vi "DecodeTDCData.vi"(11 "Buff":u32[](array[numeric])) -> (0 "Event Counter":u32, 2 "Error Read Value":u32 format="%.0x", 3 "Array":T1(array[cluster]))   [LabVIEW 2014]
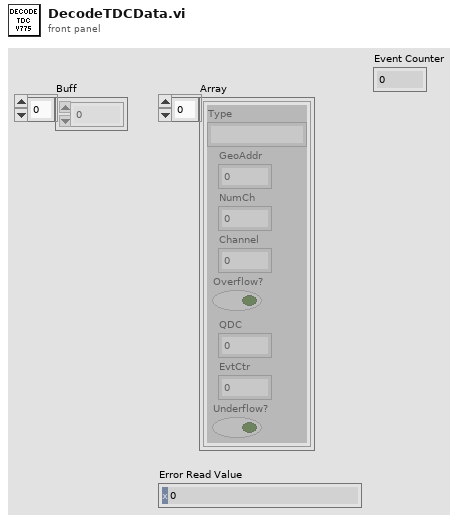
[diagram p1: front panel]
types:
  T1 = cluster{"Type":string, "GeoAddr":u8, "NumCh":u8, "Channel":u8, "Overflow?":bool, "QDC":u16, "EvtCtr":u32, "Underflow?":bool}[]
  T2 = cluster{"Type":string, "GeoAddr":u8, "NumCh":u8, "Channel":u8, "Overflow?":bool, "QDC":u16, "EvtCtr":u32, "Underflow?":bool}
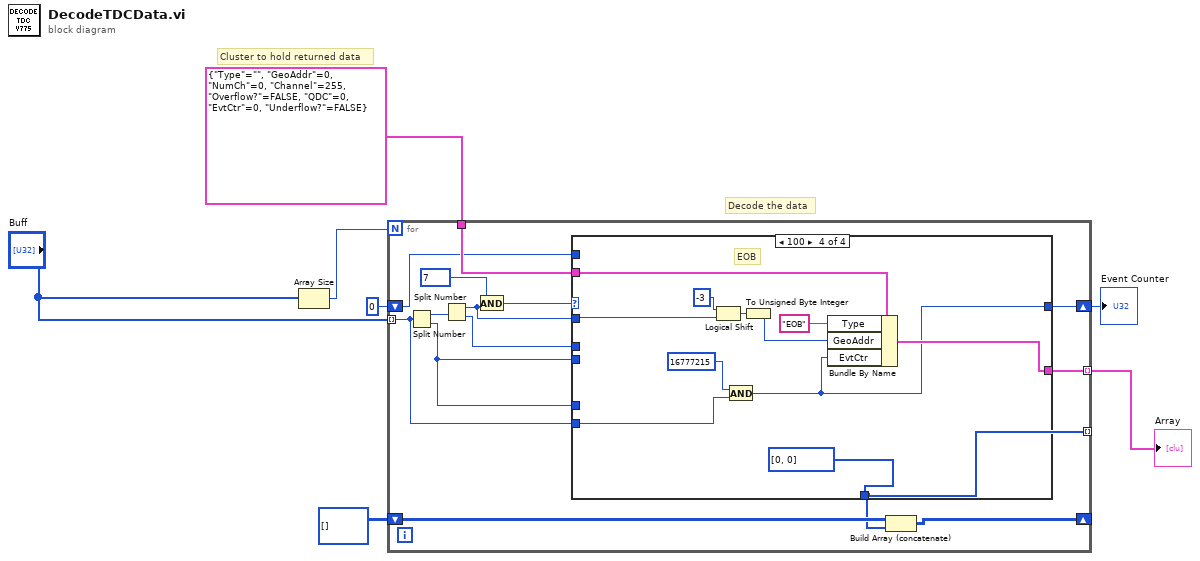
[diagram p0: block diagram]
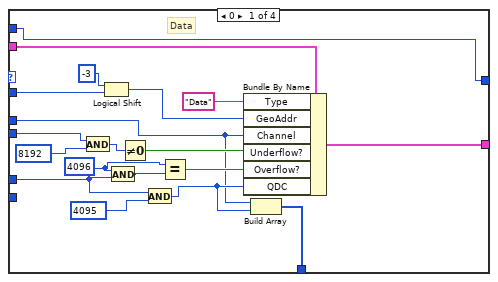
[diagram p2: hidden frame]
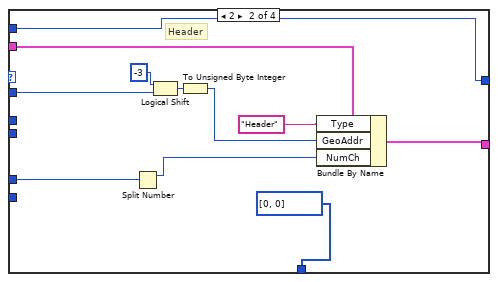
[diagram p3: hidden frame]
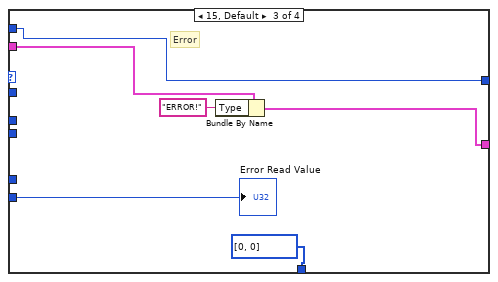
[diagram p4: hidden frame]
diagram:
  # "Decode the data"
  # "Cluster to hold returned data"
  n1 = Array Size(array="Buff") -> (size(s)=w3:i32)
  n2 = for {
    N: w3 -> [_]
    tunnel: "Buff" -> [w16] mode=indexing
    tunnel: T2 {"Type"="", "GeoAddr"=0, "NumCh"=0, "Channel"=255, "Overflow?"=FALSE, "QDC"=0, "EvtCtr"=0, "Underflow?"=FALSE} -> [w18]
    tunnel: [w14] -> w5 mode=indexing
    tunnel: [w12] -> _ mode=indexing
    shift-right: [w11] -> _
    shift-left: u32[][] [] -> [w13]
    shift-right: [w9] -> w1
    shift-left: u32 0 -> [w8]
    n3 = Split Number(x=w16) -> (hi(x)=w21:u16, lo(x)=w10:u16)
    n4 = Split Number(x=w21) -> (hi(x)=w17:u8, lo(x)=w15:u8)
    n5 = And(x=u8 7, y=w17) -> (x .and. y?=w19:u8)
    n6 = case shown="100" w19 {
      tunnel: w18 -> [w40 w47 w57 w68]
      tunnel: w17 -> [w37 w51 _ w64]
      tunnel: w10 -> [w26 w48 _ _]
      tunnel: w16 -> [_ _ w55 w62]
      tunnel: w15 -> [w28 _ _ _]
      tunnel: [w32 w43 w54 w60] -> w14
      tunnel: [w29 u32[] [0, 0] ("Buff") u32[] [0, 0] ("Buff") u32[] [0, 0] ("Buff")] -> w12
      tunnel: w10 -> [w23 _ _ _]
      tunnel: [w22 w41 w52 w58] -> w9
      tunnel: w8 -> [w22 w41 w52 _]
      frame 0 {
        w24 = u16 4096 ("y")
        # "Data"
        n7 = And(x=w23, y=u16 8192) -> (x .and. y?=w27:u16)
        n8 = Logical Shift(y=i16 -3, x=w37) -> (x << y=w34:u8)
        n9 = And(x=w24, y=w26) -> (x .and. y?=w25:u16)
        n10 = Not Equal To 0?(x=w27) -> (x != 0?=w35:bool)
        n11 = And(x=w26, y=u16 4095) -> (x .and. y?=w30:u16)
        n12 = Equal?(x=w24, y=w25) -> (x = y?=w31:bool)
        n13 = Bundle By Name(cluster=w40, "Type"="Data", "GeoAddr"=w34, "Channel"=w28, "Underflow?"=w35, "Overflow?"=w31, "QDC"=w30) -> (w32:T2)
        n14 = Build Array(w28, w30) -> (w29:u16[])
      }
      frame 2 {
        # "Header"
        n15 = Split Number(x=w48) -> (hi(x)=w44:u8)  [unwired: 1 out]
        n16 = Logical Shift(y=i16 -3, x=w51) -> (x << y=w49:u8)
        n17 = To Unsigned Byte Integer(number=w49) -> (unsigned 8bit integer=w45:u8)
        n18 = Bundle By Name(cluster=w47, "Type"="Header", "GeoAddr"=w45, "NumCh"=w44) -> (w43:T2)
      }
      frame 15, Default {
        # "Error"
        n19 = Bundle By Name(cluster=w57, "Type"="ERROR!") -> (w54:T2)
        "Error Read Value" <- w55
      }
      frame 4 {
        # "EOB"
        n20 = Logical Shift(y=i16 -3, x=w64) -> (x << y=w66:u8)
        n21 = And(x=u32 16777215, y=w62) -> (x .and. y?=w58:u32)
        n22 = To Unsigned Byte Integer(number=w66) -> (unsigned 8bit integer=w63:u8)
        n23 = Bundle By Name(cluster=w68, "Type"="EOB", "GeoAddr"=w63, "EvtCtr"=w58) -> (w60:T2)
      }
    }
    n24 = Build Array (concatenate)(w13, w12) -> (w11:u32[][])
  }
  "Array" <- w5
  "Event Counter" <- w1
